vi "pad string.vi"(8 "error in (no error)":errorcluster, 9 "string size":u16, 10 "input string":string, 11 "Log File in":refnum<class "Events Log File.lvclass">) -> (0 "error out":errorcluster, 2 "output string":string, 3 "Log File out":refnum<class "Events Log File.lvclass">)   [LabVIEW 2018, in "Events Log File.lvclass"]
uses:
  Events Log File.lvclass
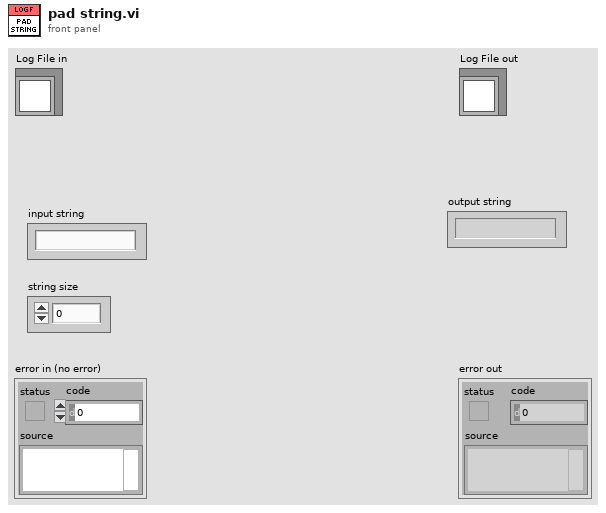
[diagram p1: front panel]
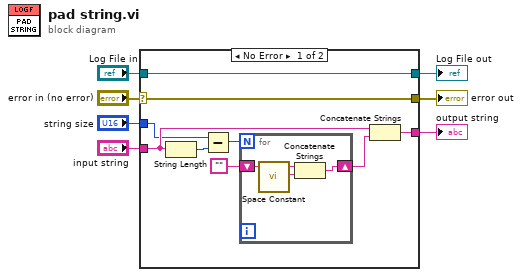
[diagram p0: block diagram]
diagram:
  n1 = case shown="No Error" "error in (no error)" {
    selector: "error in (no error)" -> [w15 w21]
    tunnel: [w15 w21] -> w6
    tunnel: [w16 w20] -> w4
    tunnel: "Log File in" -> [w16 w20]
    tunnel: "input string" -> [w10 _]
    tunnel: [w9 _] -> w2
    tunnel: "string size" -> [w8 _]
    frame No Error {
      n2 = String Length(string=w10) -> (length=w14:i32)
      n3 = Subtract(x=w8, y=w14) -> (x-y=w12:i32)
      n4 = for {
        N: w12 -> [_]
        shift-right: [w18] -> w11
        shift-left: "" -> [w19]
        n5 = call <vilib>:"Space Constant.vi"() -> ("String"=w17:string)
        n6 = Concatenate Strings(w19, w17) -> (w18:string)
      }
      n7 = Concatenate Strings(w10, w11) -> (w9:string)
    }
    frame Error {
    }
  }
  "error out" <- w6
  "Log File out" <- w4
  "output string" <- w2
